vi "CoefficientOverlays.vi"(6 "plotInfoArray":T1(array[cluster]), 7 "\"At\" location":T4={"XcoordSys"="graph", "YcoordSys"="graph", "Xvalue"=0.05, "Yvalue"=0.92}, 9 "BL Targets":T2[](array[typedef]) {"n" min=0.02 max=0.5 step=0.01 format="%.2f"}, 10 "Coefficients":cluster{"No d0":T3, "with d0":T3}, 11 "gnuplotIn":string) -> (3 "gnuplotOut":string)   [LabVIEW 2021]
uses:
  at.ctl
  PowerLaw.ctl
  BLTarget.ctl
panel:
  out "resulting string":string
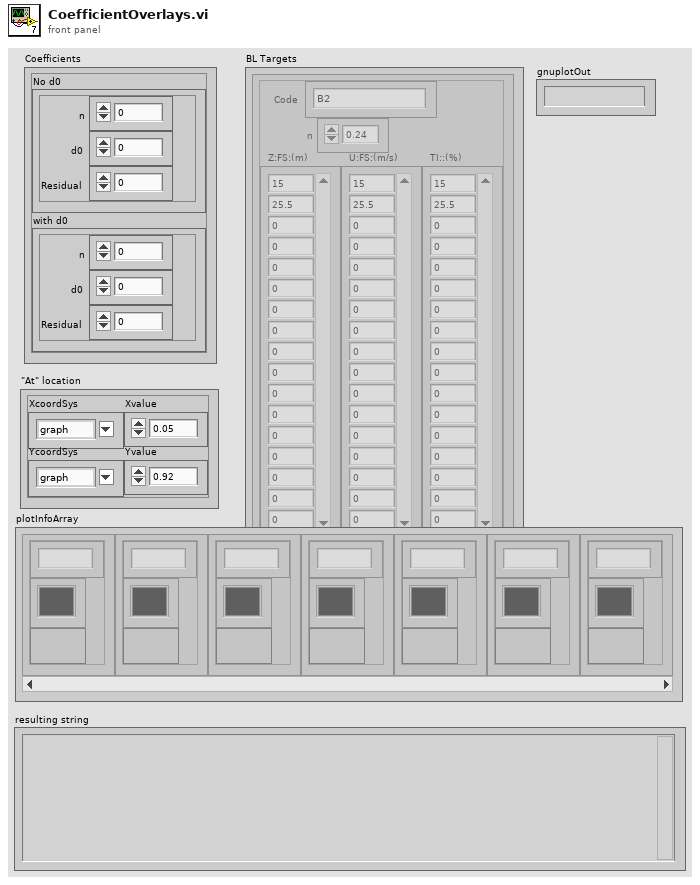
[diagram p1: front panel]
types:
  T1 = cluster{"Plot Name":string, "Plot.Plot Color":u32, "Plot.Visible?":bool}[]
  T2 = typedef "BLTarget.ctl" = cluster{"Code":string, "n":dbl, "Z:FS:(m)":dbl[], "U:FS:(m/s)":dbl[], "TI::(%)":dbl[]}
  T3 = typedef "PowerLaw.ctl" = cluster{"n":dbl, "d0":dbl, "Residual":dbl}
  T4 = typedef "at.ctl" = cluster{"XcoordSys":string, "YcoordSys":string, "Xvalue":dbl, "Yvalue":dbl}
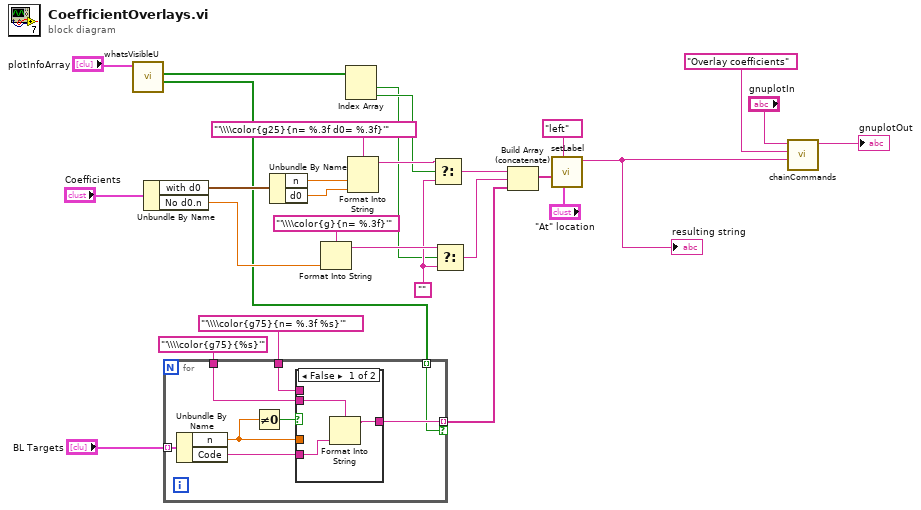
[diagram p0: block diagram]
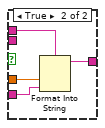
[diagram p2: hidden frame]
diagram:
  w14 = ""
  n1 = call "whatsVisibleU.vi"("UplotInfoArray"="plotInfoArray") -> ("Targets Visible"=w5:bool[], "Fits Visible"=w2:bool[])  [unwired: 8 in, 1 out]
  n2 = Unbundle By Name("Coefficients") -> ("with d0"=w20:T3, "No d0.n"=w19:dbl)
  n3 = for {
    tunnel: "'\\\\color{g75}{n= %.3f %s}'" ("format string") -> [w36]
    tunnel: [w35] -> w7 mode=indexing if=w32
    tunnel: w5 -> [w32] mode=indexing
    tunnel: "BL Targets" -> [w34] mode=indexing
    tunnel: "'\\\\color{g75}{%s}'" ("format string") -> [w29]
    n4 = Unbundle By Name(w34) -> ("n"=w30:dbl, "Code"=w33:string)
    n5 = Not Equal To 0?(x=w30) -> (x != 0?=w31:bool)
    n6 = case shown="False" w31 {
      tunnel: w36 -> [_ w43]
      tunnel: [w39 w42] -> w35
      tunnel: w30 -> [_ w41]
      tunnel: w33 -> [w37 w40]
      tunnel: w29 -> [w38 _]
      frame False {
        n7 = Format Into String(format string=w38, w37) -> (resulting string=w39:string)  [unwired: 2 in, 1 out]
      }
      frame True {
        n8 = Format Into String(format string=w43, w41, w40) -> (resulting string=w42:string)  [unwired: 2 in, 1 out]
      }
    }
  }
  n9 = Unbundle By Name(w20) -> ("n"=w28:dbl, "d0"=w26:dbl)
  n10 = Format Into String(format string="'\\\\color{g}{n= %.3f}'", w19) -> (resulting string=w17:string)  [unwired: 2 in, 1 out]
  n11 = Index Array(array=w2) -> (element #1=w3:bool, element #2=w4:bool)  [unwired: 2 in]
  n12 = Format Into String(format string="'\\\\color{g25}{n= %.3f d0= %.3f}'", w28, w26) -> (resulting string=w18:string)  [unwired: 2 in, 1 out]
  n13 = Select(t=w18, s=w4, f=w14) -> (s? t:f=w16:string)
  n14 = Select(t=w17, s=w3, f=w14) -> (s? t:f=w15:string)
  n15 = Build Array (concatenate)(w16, w15, w7) -> (w22:string[])
  n16 = call "setLabel.vi"("\"At\" location"="\"At\" location", "Justify"="left", "multilineLabel"=w22) -> ("String out"=w13:string)  [unwired: 7 in, 1 out]
  "resulting string" <- w13
  n17 = call "chainCommands.vi"("Command"=w13, "Comments"="Overlay coefficients", "StringIn"="gnuplotIn") -> ("StringOut"=→"gnuplotOut":string)  [unwired: 8 in]
